vi "LoadVK4.vi"() -> ()   [LabVIEW 2012]
uses:
  ImageHeaderType.ctl
panel:
  in  "Tab Control":T1(tab)
  in  "SaveRaw":bool
  in  "SavePics":bool
  in  "PathToVK4":path
  out "OpticalOff":u32
  out "LOoff":u32
  out "IntenOff":u32
  out "HeightOff":u32
  out "OpticalHead":T2
  out "LaserOpticalHead":T2
  out "IntensityHead":T2
  out "HeightHead":T2
  out "RGBarray":u32[][](array[numeric])
  out "Optical":picture
  out "LO":picture
  out "RGBarray2":u32[][](array[numeric])
  out "Intensity":picture
  out "IntenArray":u16[][](array[numeric])
  out "Height":picture
  out "HeightArray":u32[][](array[numeric])
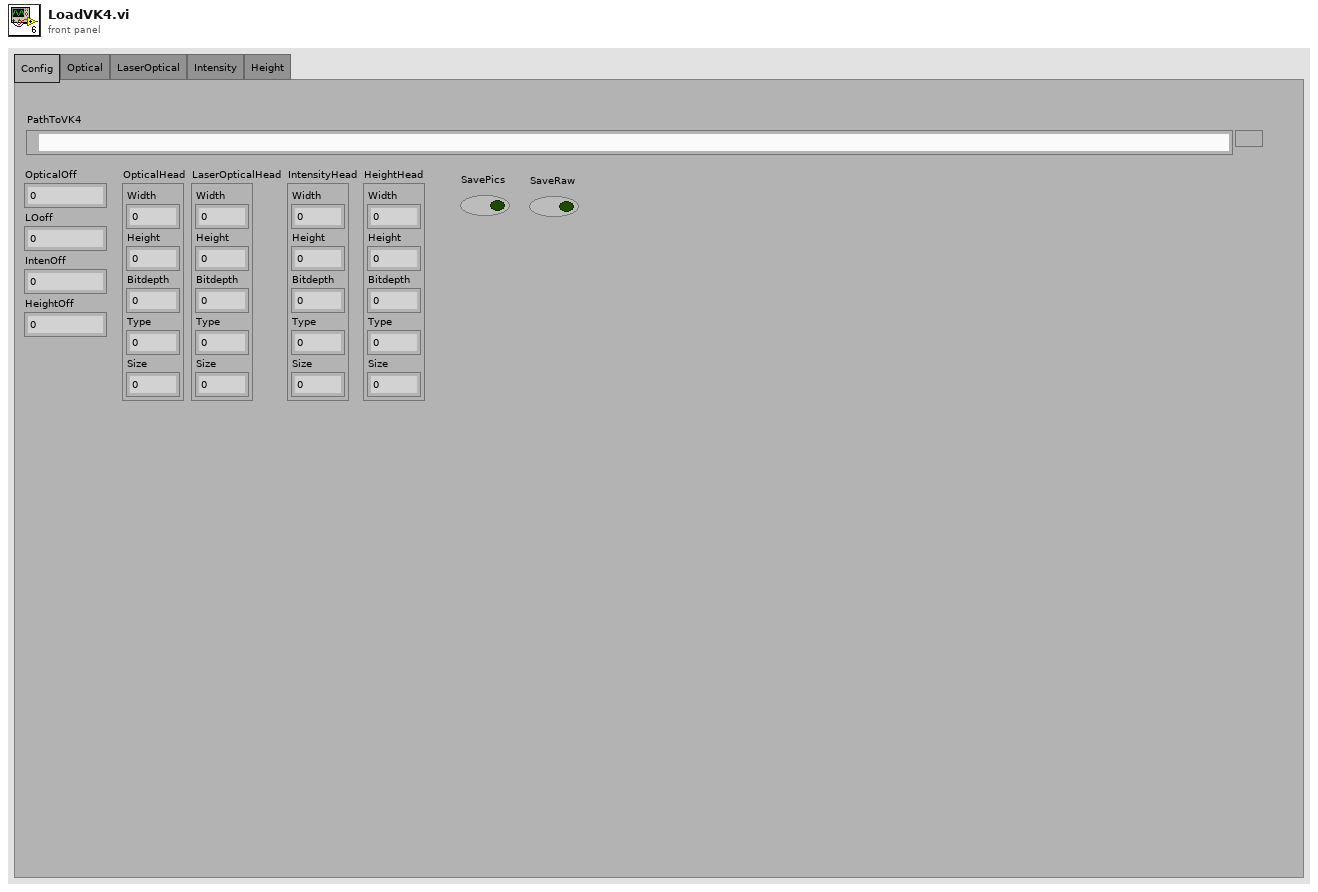
[diagram p1: front panel]
types:
  T1 = enum32{"Config", "Optical", "LaserOptical", "Intensity", "Height"}
  T2 = typedef "ImageHeaderType.ctl" = cluster{"Width":u32, "Height":u32, "Bitdepth":u32, "Type":u32, "Size":u32}
  T3 = typedef "imagedata.ctl" = cluster{"image type":i32, "image depth":i32, "image":u8[], "mask":u8[], "colors":u32[], "Rectangle":cluster{"left":i16, "top":i16, "right":i16, "bottom":i16}}
  T4 = enum16{"big-endian, network order", "native, host order", "little-endian"}
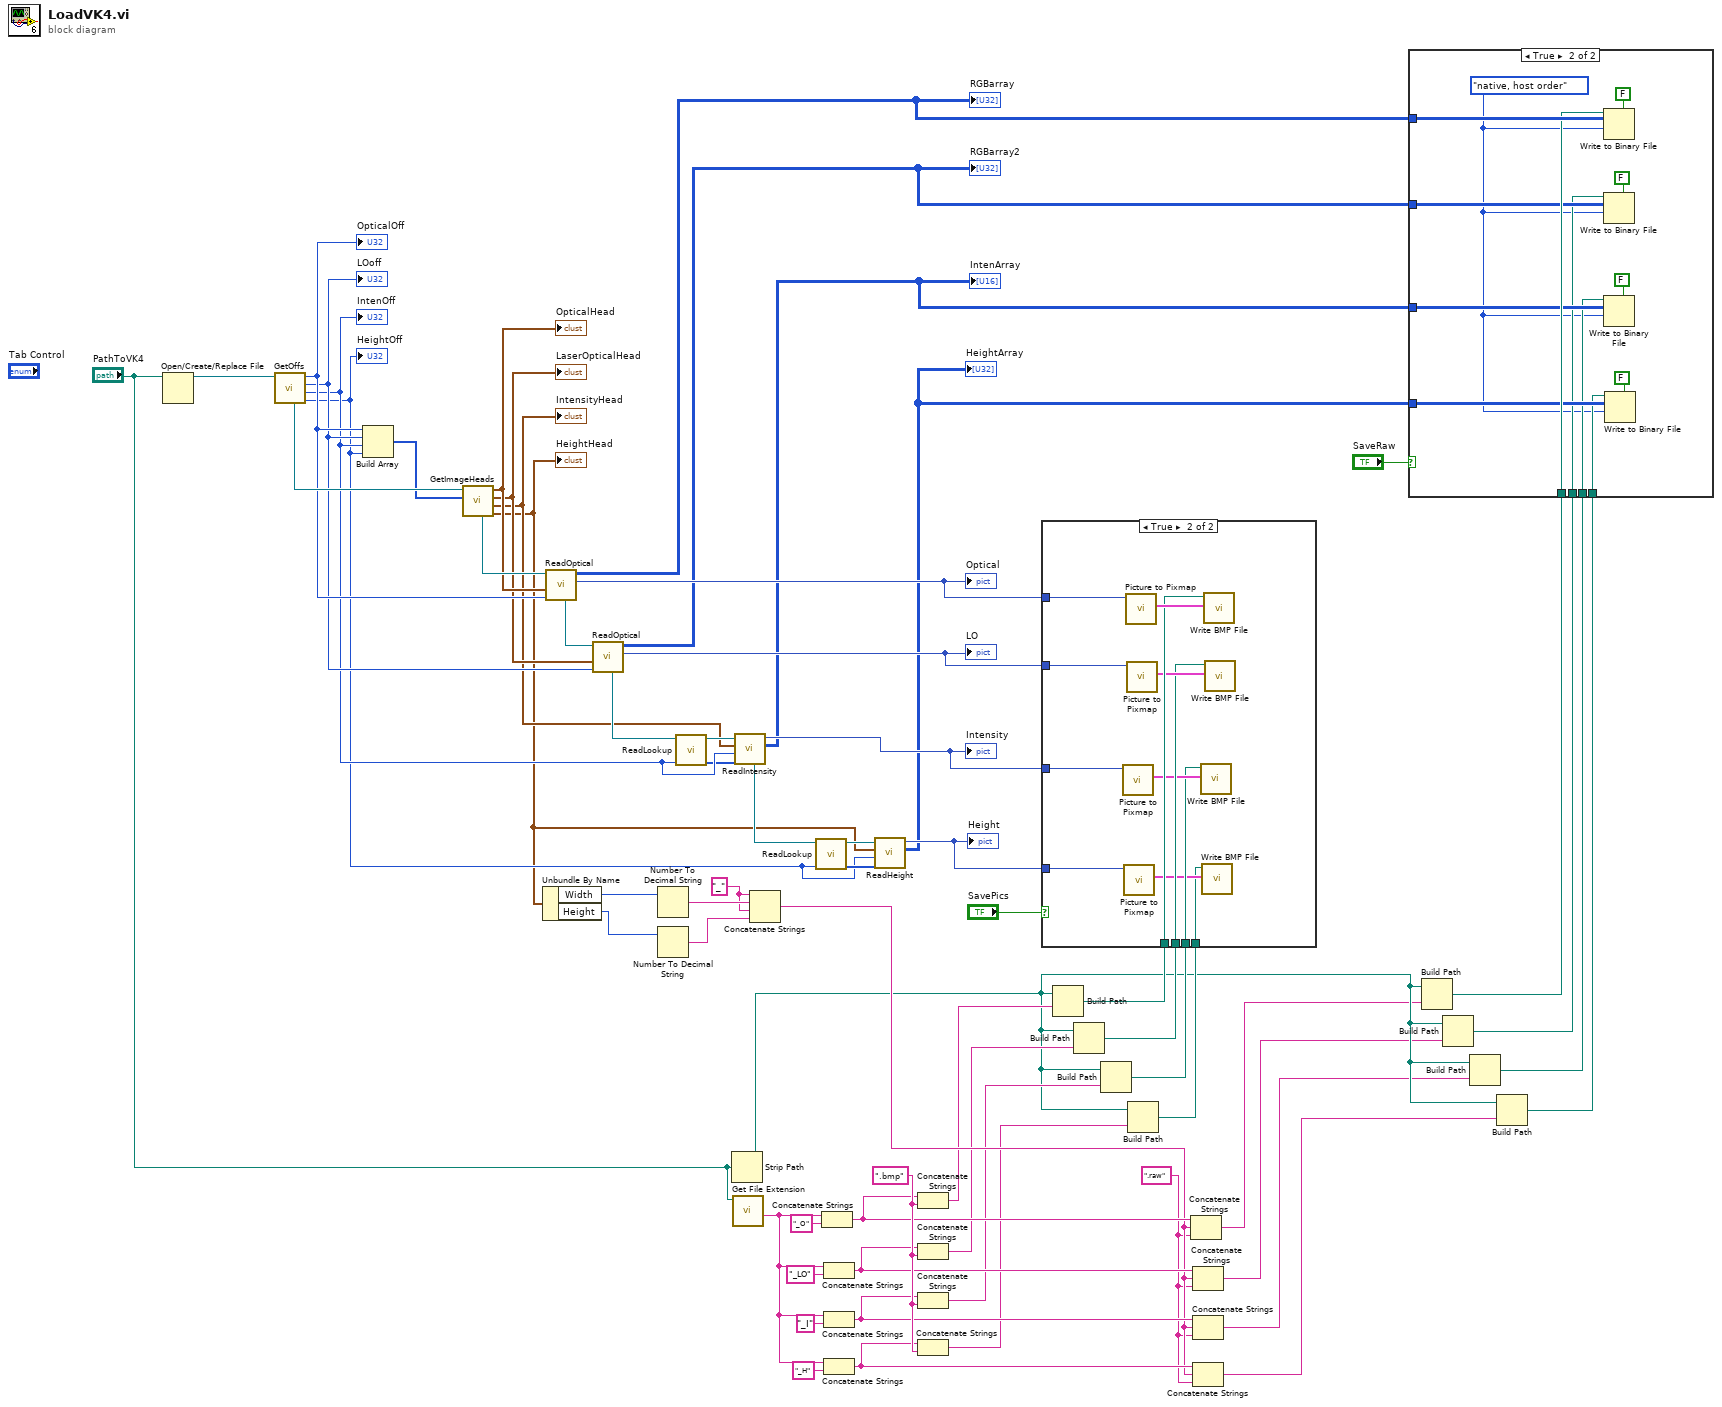
[diagram p0: block diagram]
diagram:
  w27 = ".raw" ("string")
  w29 = "_" ("string")
  w39 = ".bmp" ("string")
  n1 = Open/Create/Replace File(file path (use dialog)="PathToVK4") -> (refnum out=w64:refnum<file>)  [unwired: 5 in, 2 out]
  n2 = call "GetOffs.vi"("RefIn"=w64) -> ("HeightOff"=w47:u32, "IntenOff"=w52:u32, "LOoff"=w56:u32, "OpticalOff"=w59:u32, "RefOut"=w63:refnum<file>)  [unwired: 6 in]
  "OpticalOff" <- w59
  "LOoff" <- w56
  "IntenOff" <- w52
  "HeightOff" <- w47
  n3 = Build Array(w59, w56, w52, w47) -> (w62:u32[])
  n4 = call "GetImageHeads.vi"("Offsets"=w62, "RefIn"=w63) -> ("HeightHead"=w34:T2, "IntensityHead"=w53:T2, "LaserOpticalHead"=w57:T2, "OpticalHead"=w60:T2, "RefOut"=w61:refnum<file>)  [unwired: 5 in]
  "OpticalHead" <- w60
  "LaserOpticalHead" <- w57
  "IntensityHead" <- w53
  "HeightHead" <- w34
  n5 = Unbundle By Name(w34) -> ("Width"=w33:u32, "Height"=w32:u32)
  n6 = call "ReadOptical.vi"("OpticalOff"=w59, "OpticalHead"=w60, "RefIn"=w61) -> ("PicOut"=w26:picture, "RGBarray"=w4:u32[][], "RefOut"=w58:refnum<file>)  [unwired: 6 in]
  "RGBarray" <- w4
  "Optical" <- w26
  n7 = call "ReadOptical.vi"("OpticalOff"=w56, "OpticalHead"=w57, "RefIn"=w58) -> ("PicOut"=w23:picture, "RGBarray"=w3:u32[][], "RefOut"=w55:refnum<file>)  [unwired: 6 in]
  "LO" <- w23
  "RGBarray2" <- w3
  n8 = Number To Decimal String(number=w33) -> (decimal integer string=w31:string)  [unwired: 1 in]
  n9 = Number To Decimal String(number=w32) -> (decimal integer string=w30:string)  [unwired: 1 in]
  n10 = call "ReadLookup.vi"("IntenOff"=w52, "RefIn"=w55) -> ("Lookup"=w51:u32[], "RefOut"=w54:refnum<file>)  [unwired: 8 in]
  n11 = Strip Path(path="PathToVK4") -> (stripped path=w13:path)  [unwired: 1 out]
  n12 = call <vilib>:"Get File Extension.vi"("file"="PathToVK4") -> ("filename without extension"=w41:string)  [unwired: 7 in, 3 out]
  n13 = call "ReadIntensity.vi"("Lookup"=w51, "IntenOff"=w52, "IntensityHead"=w53, "RefIn"=w54) -> ("Intensity"=w2:u16[][], "IntenPic"=w20:picture, "RefOut"=w48:refnum<file>)  [unwired: 5 in]
  "Intensity" <- w20
  "IntenArray" <- w2
  n14 = Concatenate Strings(w29, w31, w29, w30) -> (w28:string)
  n15 = call "ReadLookup.vi"("IntenOff"=w47, "RefIn"=w48) -> ("Lookup"=w50:u32[], "RefOut"=w49:refnum<file>)  [unwired: 8 in]
  n16 = Concatenate Strings(w41, "_O" ("string")) -> (w38:string)
  n17 = Concatenate Strings(w41, "_LO" ("string")) -> (w37:string)
  n18 = Concatenate Strings(w41, "_I" ("string")) -> (w36:string)
  n19 = Concatenate Strings(w41, "_H" ("string")) -> (w35:string)
  n20 = call "ReadHeight.vi"("Lookup"=w50, "IntenOff"=w47, "IntensityHead"=w34, "RefIn"=w49) -> ("Intensity"=w1:u32[][], "IntenPic"=w17:picture)  [unwired: 5 in, 1 out]
  "Height" <- w17
  "HeightArray" <- w1
  n21 = Concatenate Strings(w38, w39) -> (w25:string)
  n22 = Concatenate Strings(w37, w39) -> (w22:string)
  n23 = Concatenate Strings(w36, w39) -> (w19:string)
  n24 = Concatenate Strings(w35, w39) -> (w16:string)
  n25 = Build Path(base path=w13, name or relative path=w25) -> (appended path=w24:path)
  n26 = Build Path(base path=w13, name or relative path=w22) -> (appended path=w21:path)
  n27 = Build Path(base path=w13, name or relative path=w19) -> (appended path=w18:path)
  n28 = Build Path(base path=w13, name or relative path=w16) -> (appended path=w15:path)
  n29 = case shown="True" "SavePics" {
    tunnel: w26 -> [_ w76]
    tunnel: w24 -> [_ w74]
    tunnel: w23 -> [_ w72]
    tunnel: w21 -> [_ w71]
    tunnel: w20 -> [_ w69]
    tunnel: w18 -> [_ w68]
    tunnel: w17 -> [_ w67]
    tunnel: w15 -> [_ w65]
    frame False {
    }
    frame True {
      n30 = call <vilib>:"Picture to Pixmap.vi"("picture"=w69) -> ("image data"=w70:T3)  [unwired: 9 in, 1 out]
      n31 = call <vilib>:"Picture to Pixmap.vi"("picture"=w67) -> ("image data"=w66:T3)  [unwired: 9 in, 1 out]
      n32 = call <vilib>:"Picture to Pixmap.vi"("picture"=w76) -> ("image data"=w75:T3)  [unwired: 9 in, 1 out]
      n33 = call <vilib>:"Picture to Pixmap.vi"("picture"=w72) -> ("image data"=w73:T3)  [unwired: 9 in, 1 out]
      n34 = call <vilib>:"Write BMP File.vi"("image data"=w70, "path to BMP file"=w68) -> ()  [unwired: 8 in, 2 out]
      n35 = call <vilib>:"Write BMP File.vi"("image data"=w66, "path to BMP file"=w65) -> ()  [unwired: 8 in, 2 out]
      n36 = call <vilib>:"Write BMP File.vi"("image data"=w75, "path to BMP file"=w74) -> ()  [unwired: 8 in, 2 out]
      n37 = call <vilib>:"Write BMP File.vi"("image data"=w73, "path to BMP file"=w71) -> ()  [unwired: 8 in, 2 out]
    }
  }
  n38 = Concatenate Strings(w38, w28, w27) -> (w12:string)
  n39 = Concatenate Strings(w37, w28, w27) -> (w11:string)
  n40 = Concatenate Strings(w36, w28, w27) -> (w10:string)
  n41 = Concatenate Strings(w35, w28, w27) -> (w9:string)
  n42 = Build Path(base path=w13, name or relative path=w12) -> (appended path=w8:path)
  n43 = Build Path(base path=w13, name or relative path=w11) -> (appended path=w7:path)
  n44 = Build Path(base path=w13, name or relative path=w10) -> (appended path=w6:path)
  n45 = Build Path(base path=w13, name or relative path=w9) -> (appended path=w5:path)
  n46 = case shown="True" "SaveRaw" {
    tunnel: w8 -> [_ w88]
    tunnel: w7 -> [_ w80]
    tunnel: w6 -> [_ w79]
    tunnel: w5 -> [_ w78]
    tunnel: w4 -> [_ w89]
    tunnel: w3 -> [_ w83]
    tunnel: w2 -> [_ w82]
    tunnel: w1 -> [_ w81]
    frame False {
    }
    frame True {
      w77 = T4."native, host order" ("byte order (0:big-endian, network order)")
      n47 = Write to Binary File(file (use dialog)=w88, data=w89, 5:FALSE ("prepend array or string size? (T)"), 9:w77) -> ()  [unwired: 2 in, 3 out]
      n48 = Write to Binary File(file (use dialog)=w80, data=w83, 5:FALSE ("prepend array or string size? (T)"), 9:w77) -> ()  [unwired: 2 in, 3 out]
      n49 = Write to Binary File(file (use dialog)=w79, data=w82, 5:FALSE ("prepend array or string size? (T)"), 9:w77) -> ()  [unwired: 2 in, 3 out]
      n50 = Write to Binary File(file (use dialog)=w78, data=w81, 5:FALSE ("prepend array or string size? (T)"), 9:w77) -> ()  [unwired: 2 in, 3 out]
    }
  }
